vi "getConnectionPoint.vi"(0 "reference":refnum<class "RectangularNode.lvclass">, 1 "direction":refnum<class "Direction.lvclass">, 5 "error in (no error)":errorcluster) -> (14 "reference out":refnum<class "RectangularNode.lvclass">, 15 "point2D":T1 {"y" format="%.2f"; "x" format="%.2f"}, 19 "error out":errorcluster)   [LabVIEW 2016, in "RectangularNode.lvclass"]
doc: "public Point2D getConnectionPoint(Direction d)"
uses:
  <resource>/Framework/Providers/Open_GDS/UML/RectangularNode_class/RectangularNode.lvclass
  <resource>/Framework/Providers/Open_GDS/UML/Direction_class/Direction.lvclass
  <resource>/Framework/Providers/Open_GDS/UML/General/Point/Point Point2D.ctl
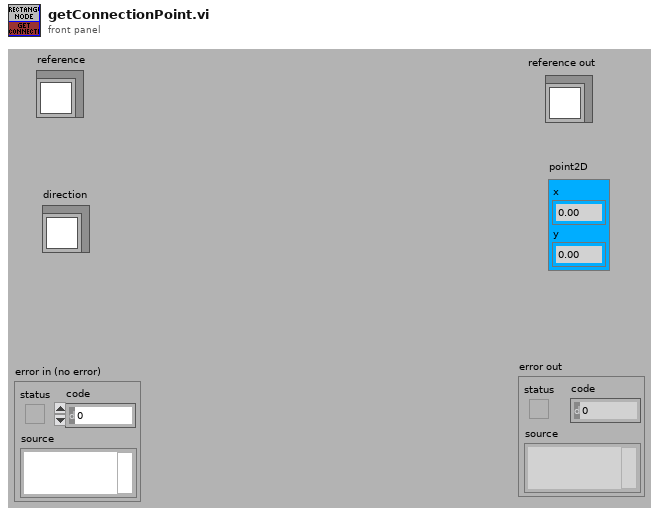
[diagram p1: front panel]
types:
  T1 = typedef "Point Point2D.ctl" = cluster{"x":dbl, "y":dbl}
  T2 = typedef "RectangularNode.lvclass/ObjectAttributes.ctl" = cluster{"bounds":T3}
  T3 = typedef "Rectangle Rectangle2D.ctl" = cluster{"x":dbl, "y":dbl, "width":dbl, "height":dbl}
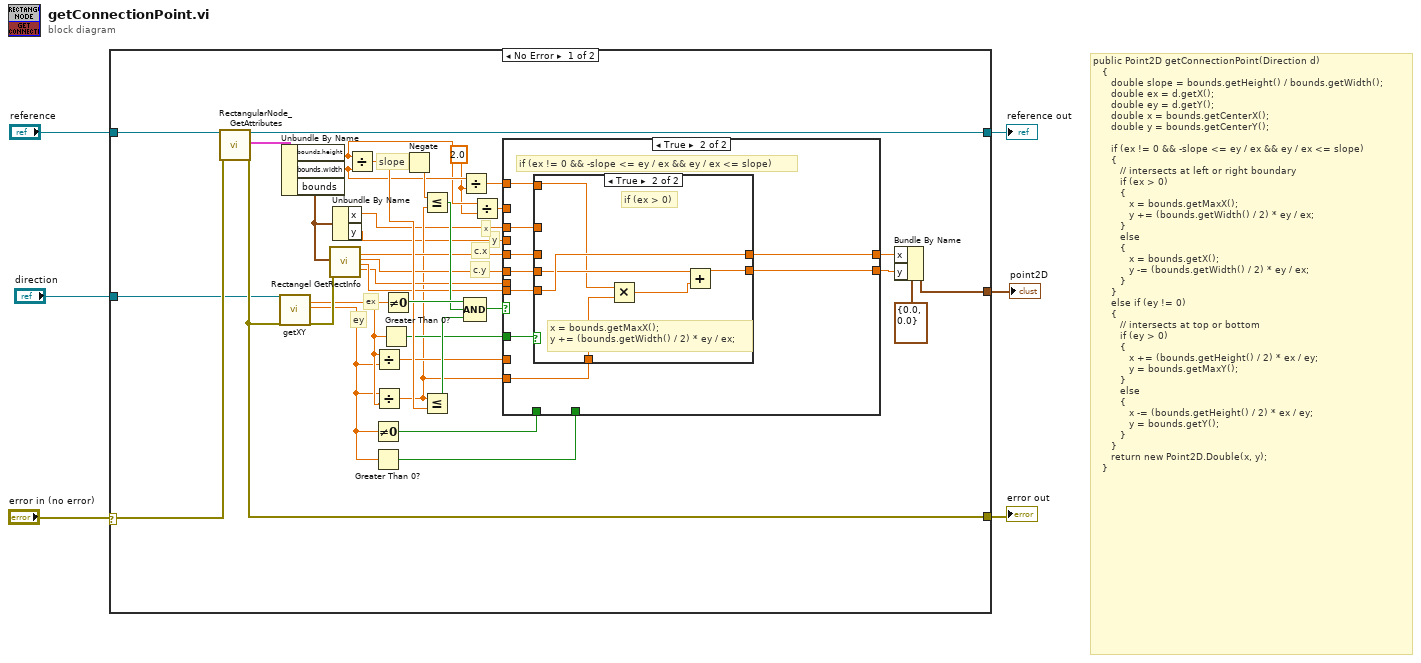
[diagram p0: block diagram]
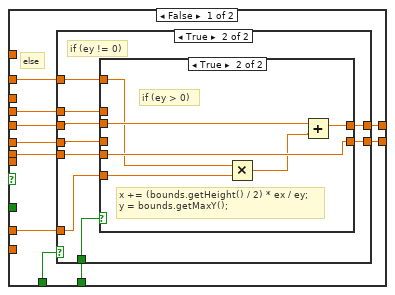
[diagram p2: hidden frame]
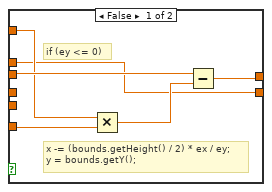
[diagram p4: hidden frame]
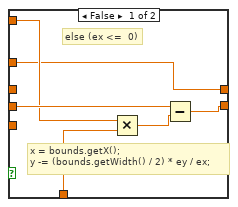
[diagram p5: hidden frame]
diagram:
  # "public Point2D getConnectionPoint(Direction d)\n   {\n      double slope = bounds.getHeight() / bounds.getWidth();\n      double ex = d.getX();\n      double ey = d.getY();\n      double x = bounds.getCenterX();\n      double y = bounds.getCenterY();\n      \n      if (ex != 0 && -slope <= ey / ex && ey / ex <= slope)\n      {  \n         // intersects at left or right boundary\n         if (ex > 0) \n         {\n            x = bounds.getMaxX();\n            y += (bounds.getWidth() / 2) * ey / ex;\n         }\n         else\n         {\n            x = bounds.getX();\n            y -= (bounds.getWidth() / 2) * ey / ex;\n         }\n      }\n      else if (ey != 0)\n      {  \n         // intersects at top or bottom\n         if (ey > 0) \n         {\n            x += (bounds.getHeight() / 2) * ex / ey;\n            y = bounds.getMaxY();\n         }\n         else\n         {\n            x -= (bounds.getHeight() / 2) * ex / ey;\n            y = bounds.getY();\n         }\n      }\n      return new Point2D.Double(x, y);\n   }"
  n1 = case shown="No Error" "error in (no error)" {
    selector: "error in (no error)" -> [w39 w97]
    tunnel: "reference" -> [w42 w98]
    tunnel: [w41 w97] -> w5
    tunnel: [w40 w98] -> w4
    tunnel: "direction" -> [w38 _]
    tunnel: [w37 _] -> w1
    frame No Error {
      w14 = 2.0 ("y")
      # "y"
      # "x"
      # "c.y"
      # "c.x"
      # "ey"
      # "ex"
      # "slope"
      n2 = call <resource>:"RectangularNode_GetAttributes.vi"("reference in"=w42, "error in (no error)"=w39) -> ("reference out"=w40:refnum<class "RectangularNode.lvclass">, "Data"=w7:T2, "error out"=w41:errorcluster)  [unwired: 1 in, 14 out]
      n3 = call <resource>:"getXY.vi"("reference"=w38, "error in (no error)"=w41) -> ("x"=w24:dbl, "y"=w22:dbl, "error out"=w36:errorcluster)  [unwired: 15 out]
      n4 = Unbundle By Name(w7) -> ("bounds.height"=w15:dbl, "bounds.width"=w17:dbl, "bounds"=w10:T3)
      n5 = call <resource>:"Rectangel GetRectInfo.vi"("bounds"=w10, "error in (no error)"=w36) -> ("centerX"=w29:dbl, "centerY"=w28:dbl, "maxX"=w20:dbl, "maxY"=w19:dbl)  [unwired: 14 out]
      n6 = Unbundle By Name(w10) -> ("x"=w9:dbl, "y"=w8:dbl)
      n7 = Divide(x=w15, y=w17) -> (x/y=w32:dbl)
      n8 = Not Equal To 0?(x=w22) -> (x != 0?=w30:bool)
      n9 = Greater Than 0?(x=w22) -> (x > 0?=w21:bool)
      n10 = Divide(x=w24, y=w22) -> (x/y=w12:dbl)
      n11 = Divide(x=w22, y=w24) -> (x/y=w11:dbl)
      n12 = Greater Than 0?(x=w24) -> (x > 0?=w23:bool)
      n13 = Not Equal To 0?(x=w24) -> (x != 0?=w35:bool)
      n14 = Negate(x=w32) -> (-x=w18:dbl)
      n15 = Less Or Equal?(x=w18, y=w11) -> (x <= y?=w33:bool)
      n16 = Less Or Equal?(x=w11, y=w32) -> (x <= y?=w31:bool)
      n17 = Divide(x=w17, y=w14) -> (x/y=w16:dbl)
      n18 = Compound Arithmetic op=AND(w35, w33, w31) -> (w34:bool)
      n19 = Divide(x=w15, y=w14) -> (x/y=w13:dbl)
      n20 = case shown="True" w34 {
        tunnel: w30 -> [w52 _]
        tunnel: w29 -> [w51 w77]
        tunnel: w28 -> [w50 w81]
        tunnel: [w49 w82] -> w27
        tunnel: [w48 w80] -> w26
        tunnel: w23 -> [_ w84]
        tunnel: w21 -> [w47 _]
        tunnel: w19 -> [w46 _]
        tunnel: w20 -> [_ w83]
        tunnel: w16 -> [_ w79]
        tunnel: w11 -> [_ w78]
        tunnel: w13 -> [w45 _]
        tunnel: w12 -> [w44 _]
        tunnel: w9 -> [_ w76]
        tunnel: w8 -> [w43 _]
        frame False {
          # "else"
          n21 = case shown="True" w52 {
            tunnel: w51 -> [w54 w60]
            tunnel: w50 -> [w53 w58]
            tunnel: [w54 w62] -> w49
            tunnel: [w53 w61] -> w48
            tunnel: w47 -> [_ w63]
            tunnel: w46 -> [_ w59]
            tunnel: w45 -> [_ w57]
            tunnel: w44 -> [_ w56]
            tunnel: w43 -> [_ w55]
            frame False {
            }
            frame True {
              # "if (ey != 0)"
              n22 = case shown="True" w63 {
                tunnel: [w68 w74] -> w62
                tunnel: [w64 w73] -> w61
                tunnel: w60 -> [w69 w75]
                tunnel: w59 -> [_ w73]
                tunnel: w58 -> [_ _]
                tunnel: w57 -> [w67 w72]
                tunnel: w56 -> [w65 w70]
                tunnel: w55 -> [w64 _]
                frame False {
                  # "x -= (bounds.getHeight() / 2) * ex / ey;\ny = bounds.getY();"
                  # "if (ey <= 0)"
                  n23 = Multiply(x=w67, y=w65) -> (x*y=w66:dbl)
                  n24 = Subtract(x=w69, y=w66) -> (x-y=w68:dbl)
                }
                frame True {
                  # "x += (bounds.getHeight() / 2) * ex / ey;\ny = bounds.getMaxY();"
                  # "if (ey > 0)"
                  n25 = Multiply(x=w72, y=w70) -> (x*y=w71:dbl)
                  n26 = Add(x=w75, y=w71) -> (x+y=w74:dbl)
                }
              }
            }
          }
        }
        frame True {
          # "if (ex != 0 && -slope <= ey / ex && ey / ex <= slope)"
          n27 = case shown="True" w84 {
            tunnel: w83 -> [_ w96]
            tunnel: [w85 w96] -> w82
            tunnel: w81 -> [w90 w95]
            tunnel: [w89 w94] -> w80
            tunnel: w79 -> [w88 w93]
            tunnel: w78 -> [w87 w92]
            tunnel: w77 -> [_ _]
            tunnel: w76 -> [w85 _]
            frame False {
              # "x = bounds.getX();\ny -= (bounds.getWidth() / 2) * ey / ex;"
              # "else (ex <=  0)"
              n28 = Multiply(x=w88, y=w87) -> (x*y=w86:dbl)
              n29 = Subtract(x=w90, y=w86) -> (x-y=w89:dbl)
            }
            frame True {
              # "x = bounds.getMaxX();\ny += (bounds.getWidth() / 2) * ey / ex;"
              # "if (ex > 0)"
              n30 = Multiply(x=w93, y=w92) -> (x*y=w91:dbl)
              n31 = Add(x=w95, y=w91) -> (x+y=w94:dbl)
            }
          }
        }
      }
      n32 = Bundle By Name(cluster=T1 {"x"=0.0, "y"=0.0} ("point2D"), "x"=w27, "y"=w26) -> (w37:T1)
    }
    frame Error {
    }
  }
  "reference out" <- w4
  "error out" <- w5
  "point2D" <- w1
